vi "Add Cursors To Graph.vi"(0 "Sunset Time":dbl format="%<%H:%M:%S>T", 5 "Sunrise Time":dbl format="%<%H:%M:%S>T", 7 "Solar Elevation Graph Ref":refnum<vi>, 9 "Postpone Time":dbl min=0.0 max=9.0 format="%<%H:%M:%S>T", 11 "Fresh Water Time":dbl min=0.0 max=12.0 format="%<%H:%M:%S>T") -> (15 "error out":errorcluster)   [LabVIEW 2024]
panel:
  out "Array":timestamp[](array[timestamp]) format="%<%.3X %x>T"
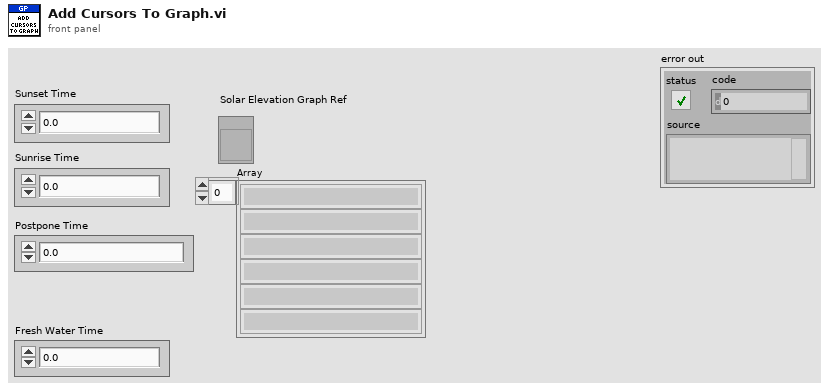
[diagram p1: front panel]
types:
  T1 = enum8{"Enabled", "Disabled", "Disabled and Grayed Out"}
  T2 = cluster{"Name":string, "Color":u32, "Style":u8, "Point Style":u8, "Name Visible":bool, "Allow Drag":bool, "Cursor Mode":u32, "Plot":i32, "Index":i32, "Position":cluster{"X":dbl, "Y":dbl}, "X Scale":u32, "Y Scale":u32, "Watch Plots":i32[], "Watch All Plots":bool, "Plot Area":i32, "Label Offset":cluster{"X":dbl, "Y":dbl}}
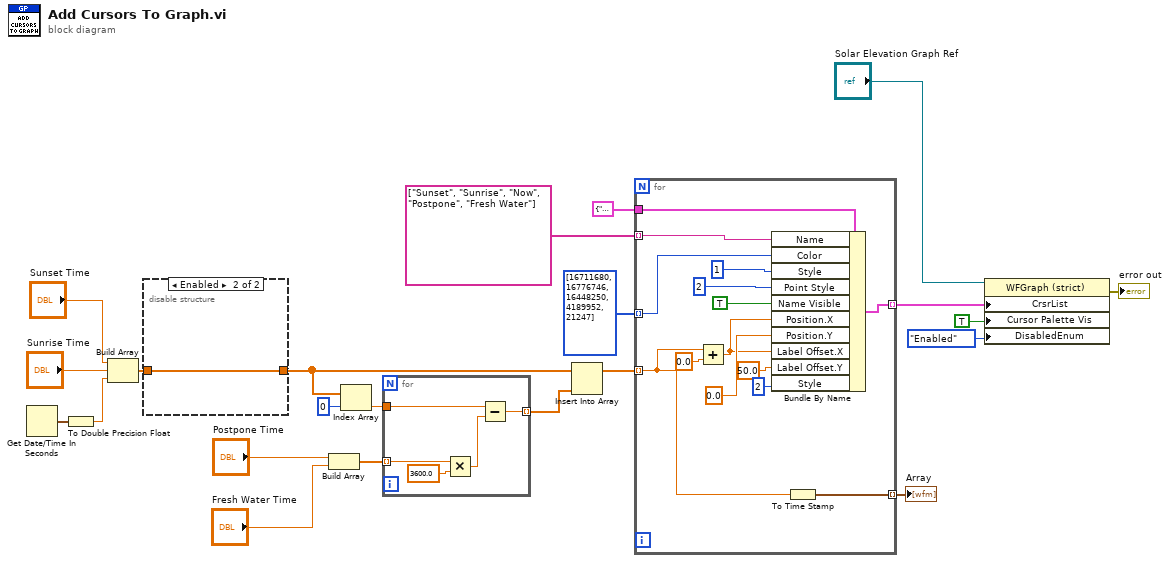
[diagram p0: block diagram]
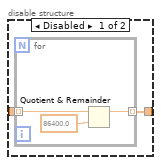
[diagram p2: hidden frame]
diagram:
  n1 = Get Date/Time In Seconds() -> (seconds since 1Jan1904=w13:timestamp)
  n2 = To Double Precision Float(number=w13) -> (double precision float=w3:dbl)
  n3 = Build Array("Sunset Time", "Sunrise Time", w3) -> (w10:dbl[])
  n4 = disable-structure shown="Enabled" {
    disable-tunnel: w10 -> [w24 w28]
    disable-tunnel: [w23 w28] -> w9
    frame Disabled {
      n5 = for {
        tunnel: w24 -> [w26] mode=indexing
        tunnel: [w25] -> w23 mode=indexing
        n6 = Quotient & Remainder(x=w26, y=86400.0) -> (x-y*floor(x/y)=w25:dbl)  [unwired: 1 out]
      }
    }
    frame Enabled {
    }
  }
  n7 = Build Array("Postpone Time", "Fresh Water Time") -> (w19:dbl[])
  n8 = Index Array(array=w9, index=0) -> (element=w7:dbl)
  n9 = for {
    tunnel: w19 -> [w31] mode=indexing
    tunnel: [w30] -> w18 mode=indexing
    tunnel: w7 -> [w29]
    n10 = Multiply(x=w31, y=3600.0) -> (x*y=w33:dbl)
    n11 = Subtract(x=w29, y=w33) -> (x-y=w30:dbl)
  }
  n12 = Insert Into Array(array=w9, new element=w18) -> (w17:dbl[])  [unwired: 1 in]
  n13 = for {
    tunnel: T2 {"Name"="", "Color"=0, "Style"=0, "Point Style"=0, "Name Visible"=FALSE, "Allow Drag"=FALSE, "Cursor Mode"=0, "Plot"=0, "Index"=0, "Position"={"X"=0.0, "Y"=0.0}, "X Scale"=0, "Y Scale"=0, "Watch Plots"=[], "Watch All Plots"=FALSE, "Plot Area"=0, "Label Offset"={"X"=0.0, "Y"=0.0}} -> [w47]
    tunnel: w17 -> [w35] mode=indexing
    tunnel: string[] ["Sunset", "Sunrise", "Now", "Postpone", "Fresh Water"] -> [w45] mode=indexing
    tunnel: u32[] [16711680, 16776746, 16448250, 4189952, 21247] -> [w44] mode=indexing
    tunnel: [w43] -> w14 mode=indexing
    tunnel: [w34] -> w1 mode=indexing
    n14 = Add(x=w35, y=0.0 ("x")) -> (x+y=w41:dbl)
    n15 = Bundle By Name(cluster=w47, "Name"=w45, "Color"=w44, "Style"=u8 1, "Point Style"=u8 2, "Name Visible"=TRUE, "Position.X"=w41, "Position.Y"=0.0, "Label Offset.X"=w41, "Label Offset.Y"=50.0, "Style"=u8 2) -> (w43:T2)
    n16 = To Time Stamp(1:w35) -> (0:w34:timestamp)
  }
  "Array" <- w1
  n17 = property on="Property Node" class="WFGraph (strict)"(reference="Solar Elevation Graph Ref", "CrsrList"=w14, "Cursor Palette Vis"=TRUE ("Cursor.Cursor Name Visible"), "DisabledEnum"=T1."Enabled" ("Disabled")) -> (error out=→"error out":errorcluster)  [unwired: 1 in, 1 out]
